vi "Get Selected Chat Message.vi"(8 "error in (no error)":errorcluster, 11 "Telegram Class in":refnum<class "Telegram Class.lvclass">) -> (0 "error out":errorcluster, 2 "Message's":string, 3 "Telegram Class out":refnum<class "Telegram Class.lvclass">)   [LabVIEW 2015, in "Telegram Library.lvlib" / "Telegram Class.lvclass"]
doc: "Created IvanLis by LabVIEW Portal\nProfile: http://labviewportal.org/memberlist.php?mode=viewprofile&u=987\neMail: IvanLisanov@gMail.com\nTelegram: https://t.me/IvanLis"
uses:
  Telegram Class.lvclass
  Telegram Class.lvclass/Telegram Class.ctl
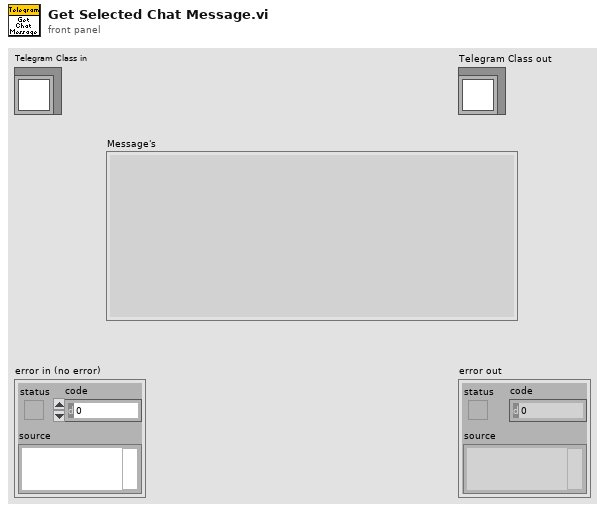
[diagram p1: front panel]
types:
  T1 = typedef "Telegram Library.lvlib/User.ctl" = cluster{"id":i64, "phone_number":string, "username":string, "last_name":string, "first_name":string}
  T2 = typedef "Telegram Library.lvlib/Message.ctl" = cluster{"id":i64, "chat_id":i64, "sender_user_id":i64, "date UTC":timestamp, "content_text":string}
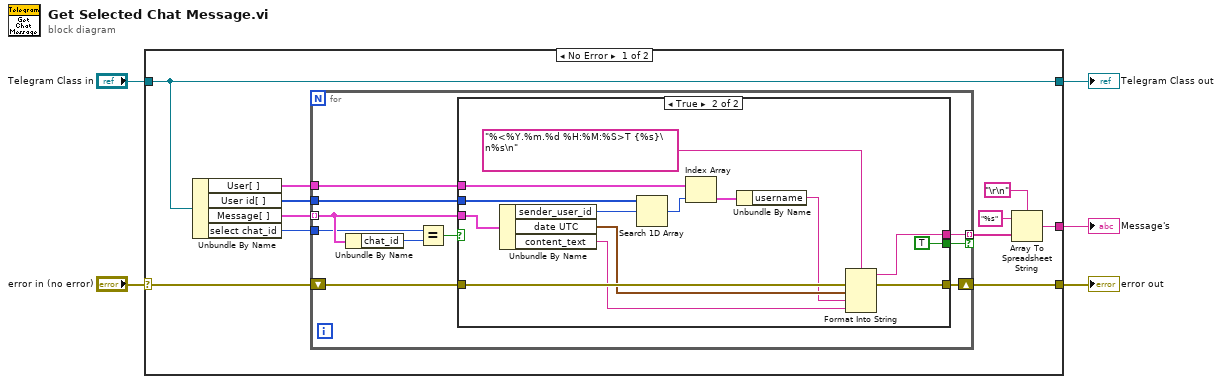
[diagram p0: block diagram]
diagram:
  n1 = case shown="No Error" "error in (no error)" {
    selector: "error in (no error)" -> [w8 w43]
    tunnel: [w14 w43] -> w4
    tunnel: [w9 w42] -> w2
    tunnel: "Telegram Class in" -> [w9 w42]
    tunnel: [w10 _] -> w1
    frame No Error {
      n2 = Unbundle By Name(w9) -> ("User[ ]"=w15:T1[], "User id[ ]"=w16:i64[], "Message[ ]"=w7:T2[], "select chat_id"=w6:i64)
      n3 = for {
        tunnel: w7 -> [w21] mode=indexing
        tunnel: w16 -> [w26]
        tunnel: w15 -> [w25]
        shift-right: [w23] -> w14
        shift-left: w8 -> [w24]
        tunnel: [w22] -> w13 mode=indexing if=w17
        tunnel: w6 -> [w20]
        n4 = Unbundle By Name(w21) -> ("chat_id"=w19:i64)
        n5 = Equal?(x=w20, y=w19) -> (x = y?=w18:bool)
        n6 = case shown="True" w18 {
          tunnel: w26 -> [_ w41]
          tunnel: w25 -> [_ w39]
          tunnel: w24 -> [w27 w37]
          tunnel: [w27 w36] -> w23
          tunnel: [_ w30] -> w22
          tunnel: w21 -> [_ w29]
          tunnel: [_ TRUE] -> w17
          frame False {
          }
          frame True {
            n7 = Unbundle By Name(w29) -> ("sender_user_id"=w40:i64, "date UTC"=w32:timestamp, "content_text"=w34:string)
            n8 = Search 1D Array(1D array=w41, element=w40) -> (index of element=w38:i32)  [unwired: 1 in]
            n9 = Index Array(array=w39, index=w38) -> (element=w35:T1)
            n10 = Unbundle By Name(w35) -> ("username"=w31:string)
            n11 = Format Into String(format string="%<%Y.%m.%d %H:%M:%S>T {%s}\n%s\n", error in=w37, w32, w31, w34) -> (resulting string=w30:string, error out=w36:errorcluster)  [unwired: 1 in]
          }
        }
      }
      n12 = Array To Spreadsheet String(delimiter (Tab)="\r\n", array=w13, 3:"%s" ("format string")) -> (spreadsheet string=w10:string)
    }
    frame Error {
    }
  }
  "error out" <- w4
  "Telegram Class out" <- w2
  "Message's" <- w1
